vi "module information (DAQmx).vi"(8 "error in":errorcluster, 11 "IP address (localhost)":string) -> (0 "error out":errorcluster, 1 "number of slots":i32, 2 "module information":T1[](array[typedef]) {"product ID" format="%.0x"})   [LabVIEW 2014, in "SMI.lvlib" / "C Series Module.lvclass"]
uses:
  C Series Module.lvclass
  Module/module information.ctl
  <vilib>/nisyscfg/Filter Mode.ctl
  <vilib>/nisyscfg/Close (Hardware).vi
  <vilib>/nisyscfg/Close (Filter).vi
  <vilib>/nisyscfg/Close (System).vi
  Module/Module.lvclass
  <resource>/objmgr/niflexriosae.rc
  <vilib>/nisyscfg/nisyscfg.lvlib
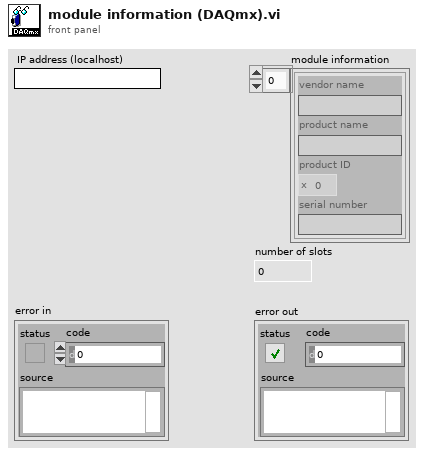
[diagram p1: front panel]
types:
  T1 = typedef "SMI.lvlib/Module.lvclass/module information.ctl" = cluster{"vendor name":string, "product name":string, "product ID":u16, "serial number":string}
  T2 = typedef "nisyscfg.lvlib/Filter Mode.ctl" = i32
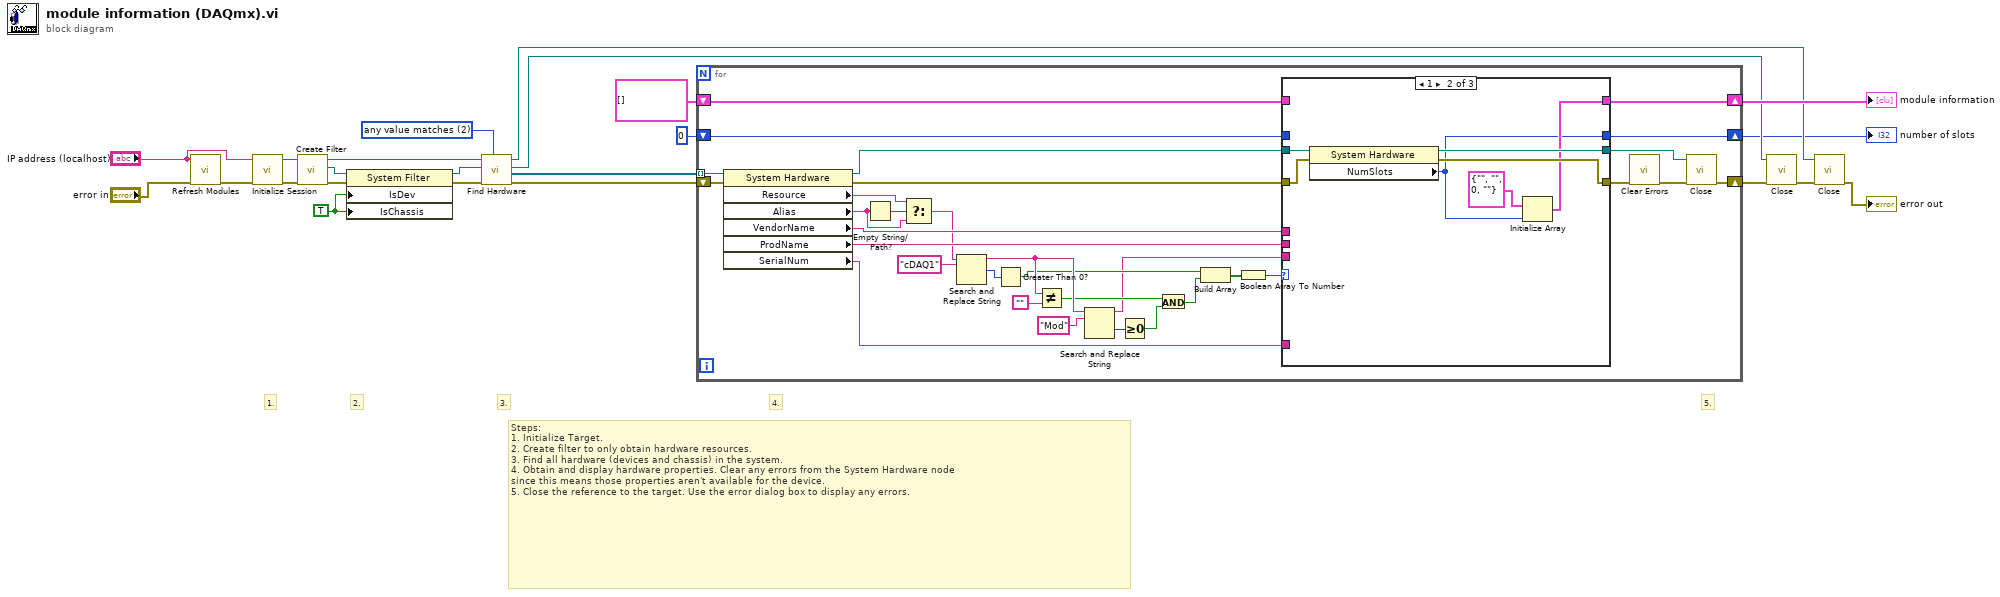
[diagram p0: block diagram]
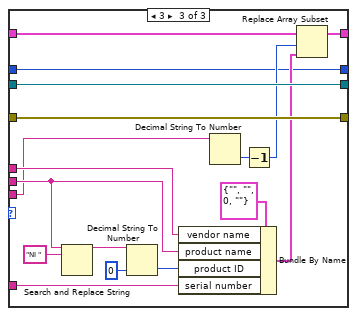
[diagram p3: hidden frame]
diagram:
  w12 = T2 2 items=["all values match"=1, "any value matches"=2, "values do not match"=3, "all properties exist"=4] ("filter mode (all values match)")
  w7 = TRUE ("Is Chassis")
  # "2."
  # "5."
  # "4."
  # "3."
  # "1."
  # "Steps:\n1. Initialize Target.\n2. Create filter to only obtain hardware resources.\n3. Find all hardware (devices and chassis) in the system.\n4. Obtain and display hardware properties. Clear any errors from the System Hardware node\nsince this means those properties aren't available for the device. \n5. Close the reference to the target. Use the error dialog box to display any errors."
  n1 = call <vilib>:"Refresh Modules.vi"("error in (no error)"="error in", "target address (localhost)"="IP address (localhost)") -> ("error out"=w1:errorcluster)  [unwired: 9 in]
  n2 = call <vilib>:"Initialize Session.vi"("error in (no error)"=w1, "Target (localhost)"="IP address (localhost)") -> ("error out"=w14:errorcluster, "Session out"=w17:refnum<k21>)  [unwired: 8 in]
  n3 = call <vilib>:"Create Filter.vi"("error in (no error)"=w14, "Session in"=w17) -> ("error out"=w19:errorcluster, "Filter out"=w18:refnum<k20>, "Session out"=w16:refnum<k21>)  [unwired: 7 in]
  n4 = property class="System Filter"(reference=w18, error in=w19, "IsDev"=w7, "IsChassis"=w7) -> (reference out=w13:refnum<k20>, error out=w15:errorcluster)
  n5 = call <vilib>:"Find Hardware.vi"("Filter Mode (all values match)"=w12, "error in (no error)"=w15, "Filter in"=w13, "Session in"=w16) -> ("error out"=w8:errorcluster, "Resources out"=w21:refnum<k20>[], "Filter out"=w10:refnum<k20>, "Session out"=w20:refnum<k21>)  [unwired: 4 out]
  n6 = for {
    tunnel: w21 -> [w53] mode=indexing
    shift-right: [w55] -> w9
    shift-left: w8 -> [w51]
    shift-right: [w28] -> w23
    shift-left: T1[] [] -> [w27]
    shift-right: [w25] -> w6
    shift-left: 0 ("NumSlots") -> [w24]
    n7 = property class="System Hardware"(reference=w53, error in=w51) -> (reference out=w31:refnum<k20>, error out=w32:errorcluster, "Resource"=w49:string, "Alias"=w52:string, "VendorName"=w46:string, "ProdName"=w48:string, "SerialNum"=w47:string)
    n8 = Empty String/Path?(string/path=w52) -> (empty?=w54:bool)
    n9 = Select(t=w49, s=w54, f=w52) -> (s? t:f=w44:string)
    n10 = Search and Replace String(input string=w44, search string="cDAQ1") -> (result string=w40:string, number of replacements=w43:i32)  [unwired: 6 in, 2 out]
    n11 = Greater Than 0?(x=w43) -> (x > 0?=w36:bool)
    n12 = Not Equal?(x=w40, y="") -> (x != y?=w38:bool)
    n13 = Search and Replace String(input string=w40, search string="Mod") -> (result string=w26:string, offset past replacement=w39:i32)  [unwired: 6 in, 2 out]
    n14 = Greater Or Equal To 0?(x=w39) -> (x >= 0?=w37:bool)
    n15 = And(x=w38, y=w37) -> (x .and. y?=w35:bool)
    n16 = Build Array(w36, w35) -> (w34:bool[])
    n17 = Boolean Array To Number(Boolean array=w34) -> (number=w33:u32)
    n18 = case shown="1" w33 {
      tunnel: w48 -> [_ _ w82]
      tunnel: w47 -> [_ _ w77]
      tunnel: w46 -> [_ _ w76]
      tunnel: w31 -> [w59 w66 w74]
      tunnel: w32 -> [w58 w65 w73]
      tunnel: [w59 w63 w74] -> w30
      tunnel: [w58 w62 w73] -> w29
      tunnel: [w57 w61 w70] -> w28
      tunnel: w27 -> [w57 _ w71]
      tunnel: w26 -> [_ _ w72]
      tunnel: [w56 w60 w67] -> w25
      tunnel: w24 -> [w56 _ w67]
      frame 0, Default {
      }
      frame 1 {
        n19 = property class="System Hardware"(reference=w66, error in=w65) -> (reference out=w63:refnum<k20>, error out=w62:errorcluster, "NumSlots"=w60:i32)
        n20 = Initialize Array(T1 {"vendor name"="", "product name"="", "product ID"=0, "serial number"=""} ("cRIO Module Information"), w60) -> (w61:T1[])
      }
      frame 3 {
        n21 = Search and Replace String(input string=w82, search string="NI ") -> (result string=w80:string)  [unwired: 6 in, 3 out]
        n22 = Decimal String To Number(string=w80, default (0L)=u16 0 ("product ID")) -> (number=w78:u16)  [unwired: 1 in, 1 out]
        n23 = Bundle By Name(cluster=T1 {"vendor name"="", "product name"="", "product ID"=0, "serial number"=""} ("cRIO Module Information"), "vendor name"=w76, "product name"=w82, "product ID"=w78, "serial number"=w77) -> (w68:T1)
        n24 = Decimal String To Number(string=w72) -> (number=w75:i32)  [unwired: 2 in, 1 out]
        n25 = Decrement(x=w75) -> (x-1=w69:i32)
        n26 = Replace Array Subset(array=w71, new element=w68, index=w69) -> (w70:T1[])
      }
    }
    n27 = call <vilib>:"Clear Errors.vi"("error in (no error)"=w29) -> ("error out"=w50:errorcluster)  [unwired: 5 in, 1 out]
    n28 = call-poly <vilib>:"Close.vi"("error in (no error)"=w50, "Resource in"=w30) -> ("error out"=w55:errorcluster)  [unwired: 9 in]
  }
  "module information" <- w23
  "number of slots" <- w6
  n29 = call-poly <vilib>:"Close.vi"("error in (no error)"=w9, "Filter in"=w10) -> ("error out"=w11:errorcluster)  [unwired: 9 in]
  n30 = call-poly <vilib>:"Close.vi"("error in (no error)"=w11, "Session in"=w20) -> ("error out"=→"error out":errorcluster)  [unwired: 9 in]
